vi "Untitled 2.vi"   [LabVIEW 2013, in "Generic Data Logger.lvlib"]
uses:
  Generic Data Logger.lvlib
  <instrlib>/Fluke 2625A/Fluke 2625A.lvlib
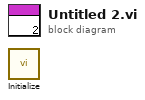
[diagram p0: block diagram]
diagram:
  n1 = call <instrlib>:"Initialize.vi"() -> ()  [unwired: 9 in, 3 out]
